vi "In the Pane.vi"(1 "Panel Bounds":T1, 2 "Reference":refnum<vi>) -> (0 "Dans le Pane":bool)   [LabVIEW 2013]
uses:
  <vilib>/Utility/miscctls.llb/LVRectTypeDef.ctl
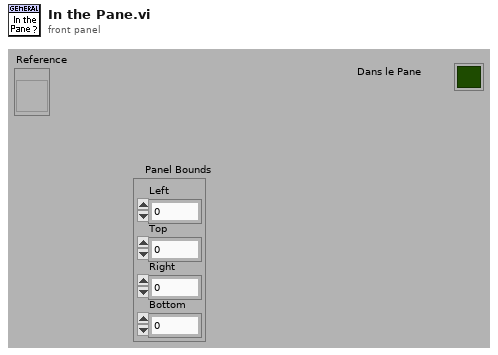
[diagram p1: front panel]
types:
  T1 = typedef "LVRectTypeDef.ctl" = cluster{"Left":i16, "Top":i16, "Right":i16, "Bottom":i16}
  T2 = typedef "LVPositionTypeDef.ctl" = cluster{"Left":i32, "Top":i32}
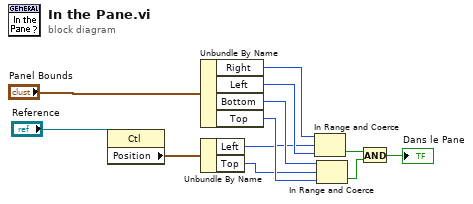
[diagram p0: block diagram]
diagram:
  n1 = property class="Ctl"(reference="Reference") -> ("Position"=w4:T2)  [unwired: 1 in, 2 out]
  n2 = Unbundle By Name("Panel Bounds") -> ("Right"=w9:i16, "Left"=w10:i16, "Bottom"=w11:i16, "Top"=w12:i16)
  n3 = Unbundle By Name(w4) -> ("Left"=w5:i32, "Top"=w6:i32)
  n4 = In Range and Coerce(upper limit=w9, x=w5, lower limit=w10) -> (In Range?=w7:bool)  [unwired: 1 out]
  n5 = In Range and Coerce(upper limit=w11, x=w6, lower limit=w12) -> (In Range?=w8:bool)  [unwired: 1 out]
  n6 = And(x=w7, y=w8) -> (x .and. y?=→"Dans le Pane":bool)
